vi "CFU_5p2_TEAM072.vi"() -> ()   [LabVIEW 2016]
uses:
  <vilib>/express/express arith-compare/Formula/XNode/ExpressFormulaBlockNode.xnode
panel:
  out "Total Resistance":dbl
  in  "Connection Type":string(combo)
  in  "R2":dbl
  in  "R1":dbl
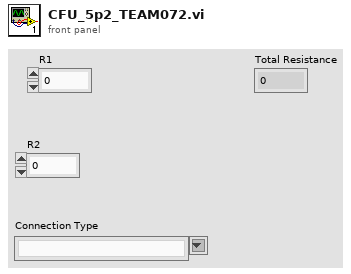
[diagram p1: front panel]
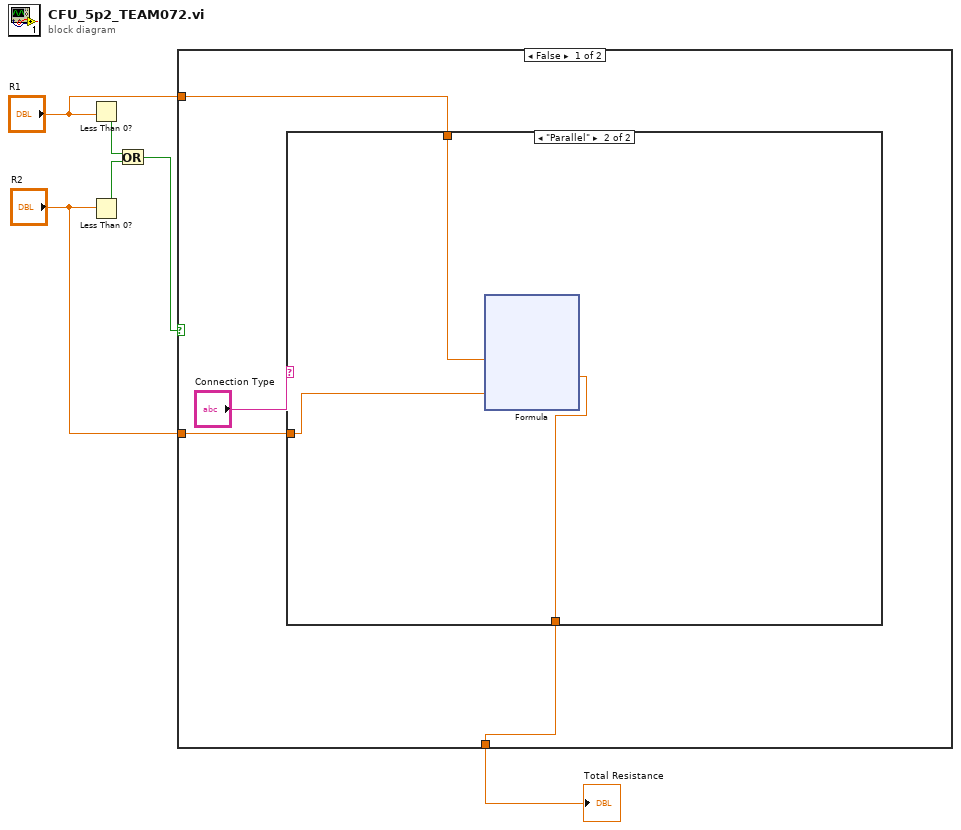
[diagram p0: block diagram]
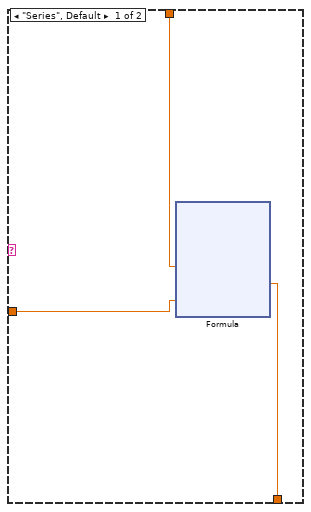
[diagram p2: hidden frame]
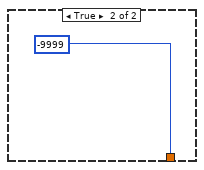
[diagram p3: hidden frame]
diagram:
  n1 = Less Than 0?(x="R1") -> (x < 0?=w5:bool)
  n2 = Less Than 0?(x="R2") -> (x < 0?=w6:bool)
  n3 = Or(x=w5, y=w6) -> (x .or. y?=w4:bool)
  n4 = case shown="False" w4 {
    tunnel: [w7 -9999] -> w3
    tunnel: "R1" -> [w9 _]
    tunnel: "R2" -> [w8 _]
    frame False {
      n5 = case shown="\"Parallel\"" "Connection Type" {
        tunnel: w9 -> [w13 w26]
        tunnel: w8 -> [w12 w25]
        tunnel: [w11 w24] -> w7
        frame "Series", Default {
          n6 = xnode "Formula"("R1"=w13, "R2"=w12) -> ("Result"=w11:dbl)  [unwired: 1 in, 1 out]
        }
        frame "Parallel" {
          n7 = xnode "Formula"("R1"=w26, "R2"=w25) -> ("Result"=w24:dbl)  [unwired: 1 in, 1 out]
        }
      }
    }
    frame True {
    }
  }
  "Total Resistance" <- w3
